vi "Wavelength Triax 550.vi"(8 "error in (no error)":errorcluster, 10 "Spectrometer Triax 550.lvclass":refnum<class "Spectrometer Triax 550.lvclass">, 11 "Wavelength in":refnum<class "Wavelength Triax 550.lvclass">) -> (0 "error out":errorcluster, 3 "Wavelength out":refnum<class "Wavelength Triax 550.lvclass">)   [LabVIEW 2017, in "Wavelength Triax 550.lvclass"]
uses:
  Wavelength Triax 550.lvclass
  C:/LabVIEW-programs/Scanners/Scanner/Scanner.lvclass
  Instruments/Spectrometer Triax 550/Spectrometer Triax 550.lvclass
  C:/LabVIEW-programs/Instruments/Utility Classes/Scannable/Scannable.lvclass
  Wavelength Triax 550.lvclass/Wavelength Triax 550.ctl
  Scanner/Scanner.lvclass
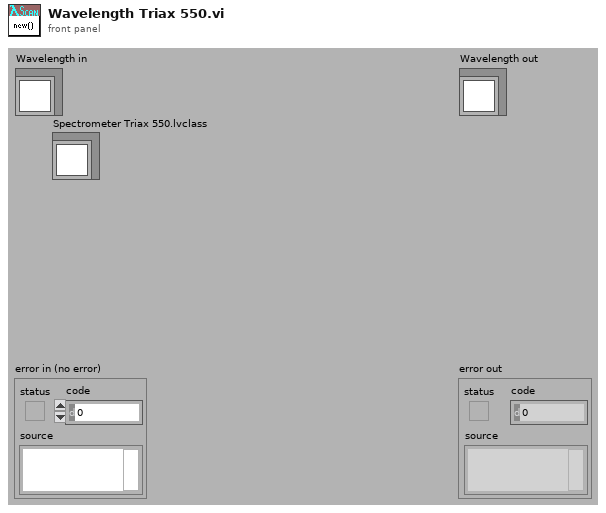
[diagram p1: front panel]
types:
  T1 = typedef "JY-SPEX-TRIAX.lvlib/Turret Position (TRIAX).ctl" = enum16{"Grating A", "Grating B", "Grating C"}
  T2 = cluster{"Turret Position":T1, "Groove Density":dbl[unit], "Blaze Wavelength":dbl[unit]}
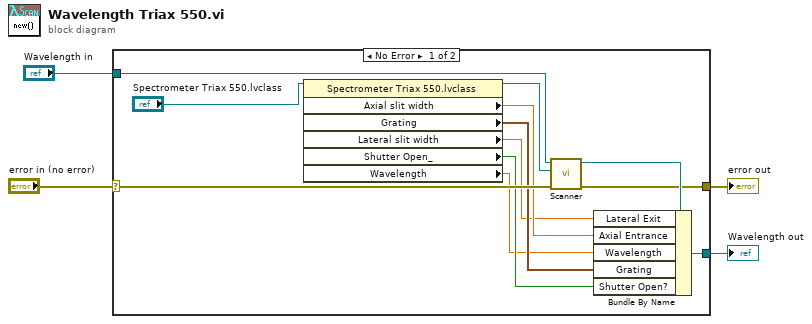
[diagram p0: block diagram]
diagram:
  n1 = case shown="No Error" "error in (no error)" {
    selector: "error in (no error)" -> [w14 w18]
    tunnel: [w13 w18] -> w3
    tunnel: [w10 w17] -> w1
    tunnel: "Wavelength in" -> [w16 w17]
    frame No Error {
      n2 = property class="Spectrometer Triax 550.lvclass"(reference="Spectrometer Triax 550.lvclass") -> (reference out=w11:refnum<class "Spectrometer Triax 550.lvclass">, "Axial slit width"=w9:dbl[unit], "Grating"=w8:T2, "Lateral slit width"=w7:dbl[unit], "Shutter Open_"=w6:bool, "Wavelength"=w5:dbl[unit])  [unwired: 1 in, 1 out]
      n3 = call "Scanner.vi"("error in (no error)"=w14, "Scannable"=w11, "Scanner.lvclass in"=w16) -> ("error out"=w13:errorcluster, "Scanner.lvclass out"=w15:refnum<class "Wavelength Triax 550.lvclass">)  [unwired: 1 in, 6 out]
      n4 = Bundle By Name(cluster=w15, "Lateral Exit"=w7, "Axial Entrance"=w9, "Wavelength"=w5, "Grating"=w8, "Shutter Open?"=w6) -> (w10:refnum<class "Wavelength Triax 550.lvclass">)
    }
    frame Error {
    }
  }
  "error out" <- w3
  "Wavelength out" <- w1
